vi "Test CONNACK packet.vi"(8 "error in (no error)":errorcluster) -> (0 "error out":errorcluster)   [LabVIEW 2013]
uses:
  source/Control Packets/CONNACK/Connect Return Code -- enum.ctl
  source/Control Packets/CONNACK/CONNACK.lvclass
  <vilib>/addons/_JKI Toolkits/Caraya/classes/Assert/Assert Equal Value_Variant.vi
  source/Control Packets/ControlPacket/ControlPacket.lvclass
  <vilib>/addons/_JKI Toolkits/Caraya/classes/Test/Test.lvclass
  <vilib>/addons/_JKI Toolkits/Caraya/classes/Assert/Assert.lvclass
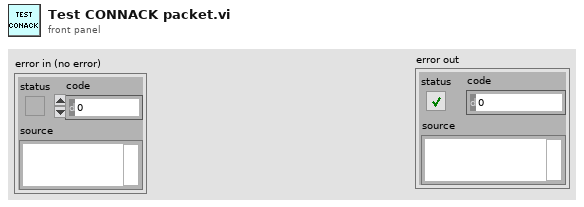
[diagram p1: front panel]
types:
  T1 = typedef "MQTT_Control_Packets.lvlib/CONNACK.lvclass/Connect Return Code -- enum.ctl" = enum16{"Connection accepted", "Unacceptable protocol version", "Identifier Rejected", "Server Unavailable", "Bad Username or Password", "Not Authorized"}
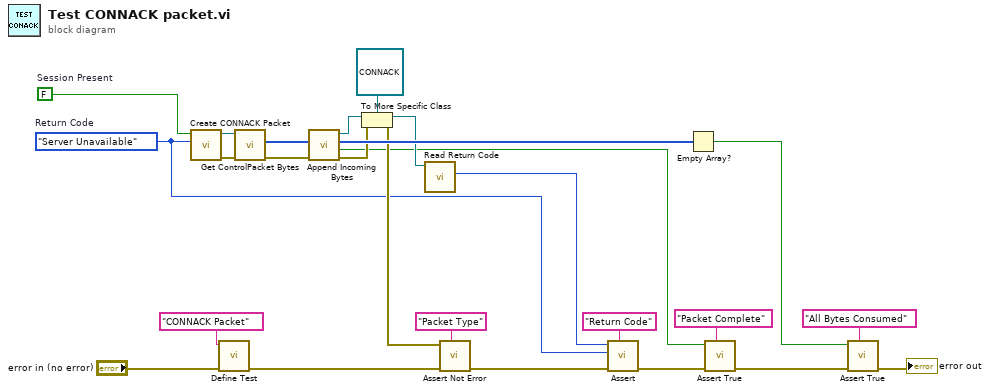
[diagram p0: block diagram]
diagram:
  w22 = FALSE  # Session Present
  w5 = Connect_Return_Code_--_enum."Server Unavailable"  # Return Code
  n1 = call "Create CONNACK Packet.vi"("Return Code"=w5, "Session Present"=w22) -> ("error out"=w20:errorcluster, "CONNACK"=w23:refnum<class "CONNACK.lvclass">)  [unwired: 8 in]
  n2 = call <vilib>:"Define Test.vi"("error in (no error)"="error in (no error)", "Label (VI Title)"="CONNACK Packet") -> ("error out"=w12:errorcluster)  [unwired: 9 in]
  n3 = call "Get ControlPacket Bytes.vi"("error in (no error)"=w20, "ControlPacket"=w23) -> ("error out"=w19:errorcluster, "Bytes Stream"=w26:u8[])  [unwired: 6 in, 2 out]
  n4 = call "Append Incoming Bytes.vi"("error in (no error)"=w19, "Incoming Packets"=w26) -> ("error out"=w18:errorcluster, "Complete Packet"=w1:bool, "Remaining Packets"=w25:u8[], "ControlPacket"=w24:refnum<class "ControlPacket.lvclass">)  [unwired: 6 in]
  n5 = To More Specific Class(target class=refnum<class "CONNACK.lvclass"> refnum ("MQTT_Control_Packets.lvlib:CONNACK.lvclass"), reference=w24, error in=w18) -> (specific class reference=w21:refnum<class "CONNACK.lvclass">, error out=w10:errorcluster)
  n6 = call "Read Return Code.vi"("CONNACK in"=w21) -> ("Return Code"=w7:T1)  [unwired: 8 in, 2 out]
  n7 = call <vilib>:"Assert Not Error.vi"("Label"="Packet Type" ("Label (VI Title)"), "error in (no error)"=w12, "Not Error?"=w10) -> ("error out"=w6:errorcluster)  [unwired: 8 in]
  n8 = call-poly <vilib>:"Assert.vi"("Label"="Return Code" ("Label (VI Title)"), "error in (no error)"=w6, "Y"=w5, "X"=w7) -> ("error out"=w3:errorcluster)  [unwired: 7 in]
  n9 = Empty Array?(array=w25) -> (empty?=w9:bool)
  n10 = call <vilib>:"Assert True.vi"("Label"="Packet Complete" ("Label (VI Title)"), "error in (no error)"=w3, "True?"=w1) -> ("error out"=w2:errorcluster)  [unwired: 8 in]
  n11 = call <vilib>:"Assert True.vi"("Label"="All Bytes Consumed" ("Label (VI Title)"), "error in (no error)"=w2, "True?"=w9) -> ("error out"=→"error out":errorcluster)  [unwired: 8 in]
